vi "UHR-Fleezers Control (host) - 12.6.vi"() -> ()   [LabVIEW 2012] (continued)
  out "X RF Frequency Limits (MHz)":T16={"Minimum"=60.0, "Maximum"=90.0, "Increment"=1.0}
  out "Y RF Frequency Limits (MHz)":T16={"Minimum"=0.0, "Maximum"=40.0, "Increment"=1.0}
  out "Y RF Amplitude Limits (%)":T16={"Minimum"=0.0, "Maximum"=50.0, "Increment"=1.0}
  in  "Manip. X?":bool=TRUE
  in  "Manip. Y?":bool
  in  "Force Manip Abort":bool
  out "Read cal error":errorcluster
  in  "DAQ Delay (ms)":u32=1000
  in  "Start Scan":bool
  in  "Scan axis":bool=TRUE
  in  "Osc. amp. (V)":dbl=5.0
  in  "Osc. center (V)":dbl=5.0
  in  "Osc. freq. (Hz) 2":dbl=1.0
  in  "MCL Mode":u16(ring) items=["Manual Positioning", "Sinusoidal Wave", "Linear Scan"]
  in  "Begin (V)":dbl
  in  "End (V)":dbl=10.0
  in  "N Points":dbl=20.0
  in  "Delay to Interlace (s)":dbl
  in  "Delayed Interlace Start":bool
  in  "Read Lateness and Rel Phase":bool=TRUE
  out "Vec Mean of T1 T2":dbl[](array[numeric])=[nan, nan]
  in  "Cal read wait (s)":u32=5
  out "Time tether formed":timestamp=timestamp(3419012832.6319866 s since 1904-01-01)
  in  "Sample Chamber Stage Serial Port":refnum<visa-resource-name>="Sample-Stage-COM1"
  in  "Chemyx Syringe Pump Serial Port":refnum<visa-resource-name>="ASRL3::INSTR"
  in  "Limit Min (MHz)":dbl=10.0 caption="Min (MHz)"
  in  "Limit Max (MHz)":dbl=16.0 caption="Max (MHz)"
  in  "Limits Enable":bool=TRUE caption="Enable"
  out "AI labels":string[](array[string])=["T1 Y", "T1 X", "T1 Sum", "T2 Y", "T2 X", "T2 Sum", "T1 FB X", "T1 FB Sum", "T2 FB X", "T2 FB Sum", "PSD Y", "PSD X", "PSD Y Sum"]
  in  "Save Trap Pos. Data":bool=TRUE
  in  "Lower Ch. Cap.":bool
  in  "Top 3 Harvard Syringe Pump Serial Port":refnum<visa-resource-name>="Top-Pump3-COM4"
  out "Database link":path
  out "connection reference":T17
  out "Trigger Signal":dbl[](graph)
  in  "Fish mask thresh":dbl=0.5
  in  "Normal (on) or masked test (off)":bool=TRUE
  in  "Stop F (pN) (mask)":dbl=1.0
  in  "Osc. freq. (Hz)":dbl=0.25
  # "External fluorescence triggering tests:"
  # "After"
  # "During"
  # "Trap On?"
  # "BD Flow ON?"
  # "Samp Flow ON?"
  # "Trap Trig. Fl.?"
  # "Zero It"
  # "Floor it\n(e.g., hp unwinding)"
  # "1"
  # "2"
  # "Fl. Down"
  # "Fl. Up"
  # "Bead sep"
  # "Trap Display:"
  # "APD Display:"
  # "Data Saving"
  # "DAQ"
  # "Trap Manipulation"
  # "Bead Calibration"
  # "Bottom Pump (#1)"
  # "Central Sample Channels"
  # "Top Pump (#3)"
  # "Rate param is ul/h\nVolume param is ul"
  # "Chemyx Pump 2"
  # "Units: \n1 = ml/m\n2 = ml/h\n3 = ul/m\n4 = ul/h"
  # "X"
  # "Y"
  # "Oscillate Set 1 freq. (debugging)"
  # "BD 1"
  # "BD 2"
  # "Amp switch 1st is disabled in the fpga!\nSeems its also frequency that needs to go first (for all boards tested so far)."
  # "AOD Raster Scan"
  # "Approx. trap separations"
  # "X"
  # "Y"
  # "FPGA\nreading"
  # "DMA\ntransfer"
  # "APD Integration Loop"
  # "APD Gates"
  # "APD 2 (Cy5)"
  # "APD 3 (Cy2)"
  # "APD 1 (Cy3)"
  # "X"
  # "2D"
  # "Y"
  # "1D"
  # "Digital Out Control"
  # "Analog Out Control (Feedback Loop)"
  # "Laser Intensity Analog Input"
  # "Operational note:\n\nUse the digital out control to adjust red laser\ntiming (fine tuning).\n\nAt the moment, the red laser analog out\ncontrol timing is identical and set by green \nlaser AO timing (in the same loop).  Otherwise\nyou can not get synchronous timing with the\ncurrent AO expansion board.\n\nSimilarly, the AI measurement is also \nsimultaneous for all three lasers (for the same\nreason).\n\nThese controls are kept for possible future\nuse."
  # "Analog Out Control (Feedback Loop)"
  # "Digital Out Control"
  # "Laser Intensity Analog Input"
  # "Operational note:\n\nThe AI measurement is simultaneous for all three lasers\n(see red laser note).\n\nThese controls are kept for possible future use."
  # "Analog Out Control (Feedback Loop)"
  # "Laser Intensity Analog Input"
  # "Digital Out Control"
  # "Total AI Rates (NOT rates/trap)"
  # "(Samples/trap x Trap Sets)"
  # "(Samples/channel x\n8 if averaging (8 channels)\n4 if no averaging)"
  # "Trap 1"
  # "Trap 2"
  # "Flour./Trap 3"
  # "External Video Window"
  # "MCL Position Debugging"
  # "Temporary Control Storage\n(these used to be somewhere else, still want to keep them)"
  # "Database config"
  # "Y"
  # "X"
  # "Trap Position Difference Limits"
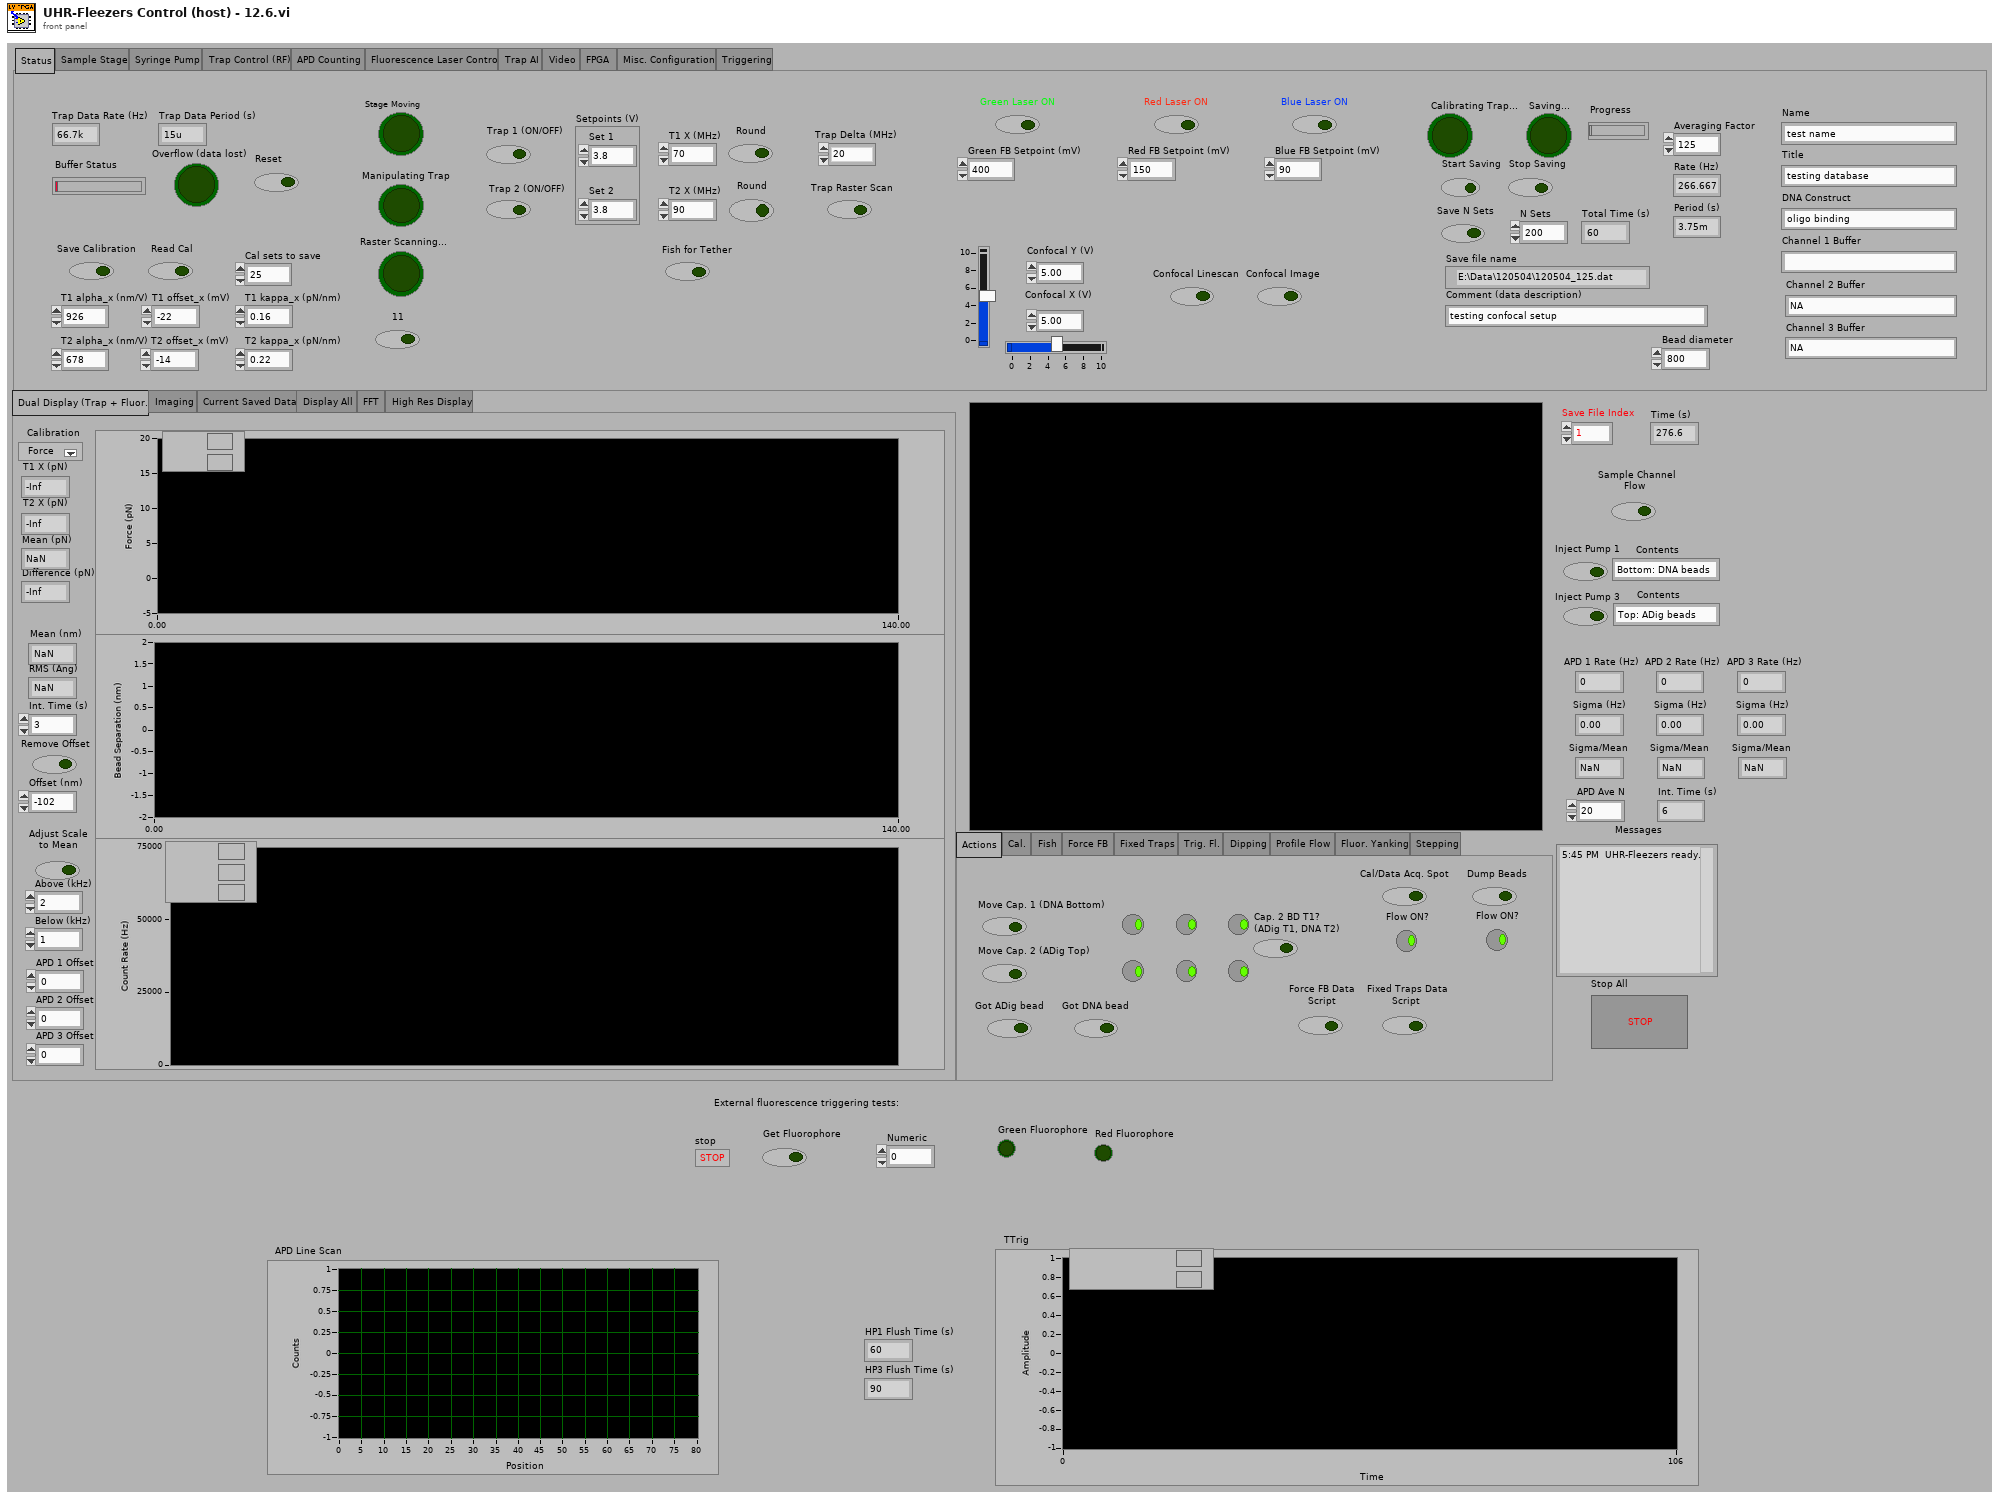
[diagram p1: front panel]
types:
  T1 = enum32{"Actions", "Cal.", "Fish", "Force FB", "Fixed Traps", "Trig. Fl.", "Dipping", "Profile Flow", "Fluor. Yanking", "Stepping"}
  T2 = typedef "IMAQ Image.ctl" = refnum<image>
  T3 = enum32{"Dual Display (Trap + Fluor.)", "Imaging", "Current Saved Data", "Display All", "FFT", "High Res Display"}
  T4 = enum32{"Status", "Sample Stage", "Syringe Pump", "Trap Control (RF)", "APD Counting", "Fluorescence Laser Control", "Trap AI", "Video", "FPGA", "Misc. Configuration", "Triggering"}
  T5 = cluster{"Pump 1":cluster{"Diameter (mm)":dbl, "Units":dbl, "Volume":dbl, "Rate":dbl}, "Pump 2":cluster{"Diameter (mm)":dbl, "Units":dbl, "Volume":dbl, "Rate":dbl}, "Pump 3":cluster{"Diameter (mm)":dbl, "Units":dbl, "Volume":dbl, "Rate":dbl}}
  T6 = enum32{"IR Laser Interlacing (Direct RF Board Control Method)", "AOD Raster Scan", "Feedback on Trap Intensity", "Feedback on Trap Position"}
  T7 = typedef "LVPoint32TypeDef.ctl" = cluster{"Horizontal":i32, "Vertical":i32}
  T8 = cluster{"Scan Range AOD (nm) 2":dbl, "Step Size AOD (nm) 2":dbl, "Scan Speed AOD (nm/s) 2":dbl, "Number of scans (AOD) 2":u16, "Label":string}[]
  T9 = cluster{"proportional gain (Kc)":i16, "integral gain (Kc*Ts/Ti)":i16, "derivative gain (Kc*Td/Ts)":i16}
  T10 = cluster{"Trap 1":fxp<+/-,16,1>, "Trap 2":fxp<+/-,16,1>}
  T11 = cluster{"proportional gain (Kc)":fxp<+/-,16,8>, "integral gain (Kc*Ts/Ti)":fxp<+/-,16,8>, "derivative gain (Kc*Td/Ts)":fxp<+/-,16,8>}
  T12 = cluster{"output high":fxp<+/-,16,1>, "output low":fxp<+/-,16,1>}
  T13 = cluster{"Set 1":fxp<+/-,16,1>, "Set 2":fxp<+/-,16,1>}
  T14 = enum32{"Main Controls", "Green laser (532 nm)", "Red laser (633 nm)", "Blue laser (473 nm)"}
  T15 = cluster{"Set 1":bool, "Set 2":bool, "Set 3":bool}
  T16 = typedef "LVMinMaxIncTypeDef.ctl" = cluster{"Minimum":dbl, "Maximum":dbl, "Increment":dbl}
  T17 = typedef "NI_Database_API.lvlib/Conn ObjectReference.ctl" = refnum<k1>
  T18 = typedef "Image Type" = u32
  T19 = typedef "nirio_resource_hc.ctl" = tag
  T20 = typedef "openfpgaref.8.6.ctl" = refnum<k20>
  T21 = enum16{"empty", "write", "read oldest (queue)", "read newest (stack)", "read all"}
  T22 = cluster{"New Image":T2, "New Image":T2, "New Image":T2, "New Image":T2, "New Image":T2}
  T23 = typedef "XDNodeRunTimeDep.lvlib/timing_clust.ctl" = cluster{"Expected End [f-1]":u64, "Actual End [f-1]":u64, "Finished Late? [f-1]":bool, "Expected End [i-1]":u64, "Actual End [i-1]":u64, "Finished Late? [i-1]":bool, "Expected Start [i]":u64, "Actual Start [i]":u64, "Expected Start [f]":u64, "Actual Start [f]":u64, "Source Name":string, "Structure Name":string, "Period":i64, "Deadline":i64, "Offset":i64, "Start":i64, "Priority":i32, "Timeout":i32, "Mode":T24, "Wakeup Reason":T25, "Error":errorcluster, "Source Type":string, "Secondary Source Type":string, "Global End Time":u64, "Global Start Time":u64, "Frame Duration":u64, "Iteration Duration":u64, "Assigned CPU":i32, "I/O Scan Engine Mode":u32}
  T24 = typedef "XDNodeRunTimeDep.lvlib/nitl_modes.ctl" = enum32{"No Change", "Process missed periods, maintain original phase", "Discard missed periods, maintain original phase", "Process missed periods, ignore original phase", "Discard missed periods, ignore original phase"}
  T25 = typedef "XDNodeRunTimeDep.lvlib/wakeup.ctl" = enum32{"Normal", "Aborted", "Asynchronous wakeup", "Timing source error", "Timed loop error", "Timeout"}
  T26 = enum32{"Status", "Sample Stage", "Syringe Pump", "Trap Control (RF)", "APD Counting", "Fluorescence Laser Control", "Trap AI", "Video", "FPGA"}
  T27 = enum32{"Status", "Sample Stage", "Syringe Pump", "Trap Control (RF)", "APD Counting", "Fluorescence Laser Control", "Trap AI", "Video", "FPGA", "Misc. Configuration"}
  T28 = enum16{"big-endian, network order", "native, host order", "little-endian"}
  T29 = enum16{"open", "replace", "create", "open or create", "replace or create", "replace or create with confirmation"}
  T30 = cluster{"Scan Range AOD (nm) 2":dbl, "Step Size AOD (nm) 2":dbl, "Scan Speed AOD (nm/s) 2":dbl, "Number of scans (AOD) 2":u16, "Label":string}
  T31 = cluster{"[0]":dbl, "[1]":dbl, "[2]":dbl, "[3]":dbl, "[4]":dbl, "[5]":dbl}
  T32 = cluster{"Diameter (mm)":dbl, "Units":dbl, "Volume":dbl, "Rate":dbl}
  T33 = cluster{"Left":i32, "Top":i32, "Width":u32, "Height":u32}
  T34 = cluster{cluster{"Left":i32, "Top":i32, "Width":u32, "Height":u32}}[]
  T35 = enum32{"Normal Display", "Dual Display (APD)", "FFT", "High Res Display"}
  T36 = cluster{"Origin Pixel":cluster{"X":sgl, "Y":sgl}, "Angle Relative to Horizontal (deg)":sgl, "Axis Reference":u32}
  T37 = typedef "Simple Grid Descriptor" = cluster{"X Step":sgl, "Y Step":sgl, "Unit":T38}
  T38 = typedef "Image Unit" = enum32{"Undefined", "Angström", "Micrometer", "Millimeter", "Centimeter", "Meter", "Kilometer", "Microinch", "Inch", "Feet", "Nautical miles", "Standard miles", "Steps"}
  T39 = cluster{"averaging mode":u16, "weighting mode":u16, "number of averages":u32}
  T40 = cluster{"dB On (F)":bool, "unwrap phase (F)":bool, "convert to degree (F)":bool}
  T41 = cluster{string, string, string, string, string, string, string, string}
  T42 = cluster{string, string, string, string, string, string, string, string, string, string, string, string}
  T43 = cluster{string, string, string, string, string, string, string, string, string, string, string, string, string}
  T44 = cluster{string, string, string, string, string, string, string, string, string, string, string, string, string, string}
  T45 = cluster{"BD 1 Frequency 1 (MHz)":dbl, "BD 1 Frequency 2 (MHz)":dbl}
  T46 = cluster{"f0":dbl, "df":dbl, "magnitude":dbl[]}[][]
  T47 = cluster{"Comment (data description)":string, "Channel 1 Buffer":string, "Channel 2 Buffer":string, "Channel 3 Buffer":string, "Title":string, "DNA Construct":string, "Bead diameter":dbl, "Name":string}
  T48 = enum32{"setting", "request", "request control", "info", "statistics", "system settings", "I/O sub system", "HRT control", "camera descriptions", "device specific data", "event sub system settings", "event sub system results", "image memory manager"}
  T49 = typedef "AviRefnum.ctl" = refnum<k1>
  T50 = typedef "imagedata.ctl" = cluster{"image type":i32, "image depth":i32, "image":u8[], "mask":u8[], "colors":u32[], "Rectangle":cluster{"left":i16, "top":i16, "right":i16, "bottom":i16}}
diagram:
  w6 = u16 10 items=["1.0"=10, "1.5"=15, "2.0"=20] ("stop bits (10: 1 bit)")
  w73 = u16 20 items=["1.0"=10, "1.5"=15, "2.0"=20] ("stop bits (10: 1 bit)")
  w76 = u16 20 items=["1.0"=10, "1.5"=15, "2.0"=20] ("stop bits (10: 1 bit)")
  w102 = u16 20 items=["1.0"=10, "1.5"=15, "2.0"=20] ("stop bits (10: 1 bit)")
  w12 = T18 2 items=["Grayscale (U8)", "Grayscale (I16)", "Grayscale (SGL)", "Complex (CSG)", "RGB (U32)", "HSL (U32)", "RGB (U64)", "Grayscale (U16)"] ("Image Type")
  w232 = 10.0 ("y")
  w231 = 32767.0 ("y")
  w247 = 6.0  # clock mult.
  w248 = 49152000.0  # TCXO frequ.
  # "What are these?"
  # "I don't think you need to do this.\nEverytime you want to adjust phase you always set this anyway.\nSince we removed the separate +/- controls.\n\nHaven't added for added fl lasers.  Should remove this code."
  # "Bottom 1 Harvard"
  # "Top 3 Harvard"
  # "Center Harvard"
  # "Bottom 1 Harvard"
  # "Top 3 Harvard"
  # "Center Harvard"
  n1 = Build Array("DIO count 1 (ticks)", "DIO count 2 (ticks)", "DIO count 3 (ticks)") -> (w153:u16[])
  n2 = xnode "Open FPGA VI Reference"("resource name"=T19 "750kHzDAQ") -> ("FPGA VI Reference Out"=w256:T20, "error out"=w255:errorcluster)  [unwired: 1 in]
  n3 = local read "AO1"() -> (w226:dbl)
  n4 = local read "AO2"() -> (w225:dbl)
  n5 = local read "Scan Increment (MHz)"() -> (w243:dbl)
  n6 = local read "Continuous MCL Scanning"() -> (w213:bool)
  n7 = local read "Fast Scan Dir"() -> (w212:bool)
  n8 = xnode "Invoke Method"("FPGA VI Reference In"=w256, "error in"=w255) -> ("FPGA VI Reference Out"=w16:T20, "error out"=w172:errorcluster)
  n9 = local read "Number of scans (MCL)"() -> (w214:u64)
  n10 = Multiply(x=w226, y=w231) -> (x*y=w228:dbl)
  n11 = Multiply(x=w225, y=w231) -> (x*y=w230:dbl)
  n12 = Divide(x=w228, y=w232) -> (x/y=w227:dbl)
  n13 = Divide(x=w230, y=w232) -> (x/y=w229:dbl)
  n14 = To Word Integer(number=w227) -> (16bit integer=w224:i16)
  n15 = To Word Integer(number=w229) -> (16bit integer=w223:i16)
  n16 = Not(x=w212) -> (.not. x?=w207:bool)
  n17 = local read "Cycles/step (MCL)"() -> (w215:u64)
  n18 = Multiply(x=w243, y=1000.0) -> (x*y=w250:dbl)
  n19 = local read "Scan steps (MCL)"() -> (w216:u64)
  n20 = local read "Desired Scan Incr (V)"() -> (w218:dbl)
  n21 = Scale By Power Of 2(n=48, x=w250) -> (x*2^n=w251:dbl)
  n22 = Unbundle By Name(cluster{"output high":i16, "output low":i16} {"output high"=3000, "output low"=0} ("FB output range 1")) -> ("output high"=w54:i16, "output low"=w53:i16)
  n23 = Multiply(x=w248, y=w247) -> (x*y=w246:dbl)
  n24 = Divide(x=w251, y=w246) -> (x/y=w245:dbl)
  n25 = local read "Setpoints (V)"() -> (w262:cluster{"Set 1":dbl, "Set 2":dbl})
  n26 = To Quad Integer(1:w245) -> (0:w242:i64)
  n27 = Divide(x=40000000.0, y="AI Count (ticks)") -> (x/y=w203:dbl)
  n28 = Multiply(x=w218, y=32767.0) -> (x*y=w220:dbl)
  n29 = local read "Trap Intensity PID Gains"() -> (w257:T9)
  n30 = local write "Trap Pos FIFO Timeout"(u16 0 ("Trap Pos FIFO Timeout")) -> ()
  n31 = local read "Number Interlace Sets"() -> (w146:u8)
  n32 = Split 1D Array(array=w153, index=w146) -> (first subarray=w155:u16[])  [unwired: 1 out]
  n33 = Add Array Elements(numeric array=w155) -> (sum=w154:u16)
  n34 = local read "# Samples/channel"() -> (w235:u32)
  n35 = local read "Number of F/B Scans (AOD)"() -> (w236:u16)
  n36 = local read "Not-Interlacing Set"() -> (w145:enum32{"Set 1", "Set 2", "Set 3"})
  n37 = To Unsigned Byte Integer(number=w145) -> (unsigned 8bit integer=w151:u8)
  n38 = Index Array(array=w153, index=w151) -> (element=w152:u16)
  n39 = local read "Feedback On/Off"() -> (w265:cluster{"Set 1":bool, "Set 2":bool})
  n40 = local read "Scan steps (AOD)"() -> (w241:u64)
  n41 = local read "All FB On/Off"() -> (w266:bool)
  n42 = local read "Cycles/step (AOD)"() -> (w240:u64)
  n43 = local write "AI rate (Hz)"(w203) -> ()
  n44 = Divide(x=w220, y=10.0) -> (x/y=w219:dbl)
  n45 = Multiply(x=w241, y=w240) -> (x*y=w239:u64)
  n46 = Unbundle By Name(w257) -> ("proportional gain (Kc)"=w58:i16, "integral gain (Kc*Ts/Ti)"=w57:i16, "derivative gain (Kc*Td/Ts)"=w56:i16)
  n47 = property on="AI Count (ticks)" class="DigNum (strict)"("Val(Sgnl)"="AI Count (ticks)") -> ()  [unwired: 2 in, 2 out]
  n48 = Multiply(x=3276.7, y=w262) -> (x*y=w261:cluster{"Set 1":dbl, "Set 2":dbl})
  n49 = To Word Integer(number=w219) -> (16bit integer=w217:i16)
  n50 = Multiply(x=w239, y=u64 2) -> (x*y=w237:u64)
  n51 = Divide(x=w203, y="FPGA Ave.") -> (x/y=w204:dbl)
  n52 = To Word Integer(number=w261) -> (16bit integer=w260:cluster{"Set 1":i16, "Set 2":i16})
  n53 = Multiply(x=w237, y=w236) -> (x*y=w234:u64)
  n54 = local read "Sets to FIFO (Traps)"() -> (w62:T15)
  n55 = local write "Ave. Rate (Hz)"(w204) -> ()
  n56 = Divide(x=w234, y=w235) -> (x/y=w233:dbl)
  n57 = Unbundle By Name(w260) -> ("Set 1"=w259:i16, "Set 2"=w258:i16)
  n58 = local read "2D or 1D Scan"() -> (w164:bool)
  n59 = local write "Data points/scans"(w234) -> ()
  n60 = local read "Scan BD"() -> (w252:bool)
  n61 = And(x=w265, y=w266) -> (x .and. y?=w264:cluster{"Set 1":bool, "Set 2":bool})
  n62 = local write "Data points/scan (f/b)"(w237) -> ()
  n63 = Reciprocal(x=w204) -> (1/x=w205:dbl)
  n64 = local read "N Acq Sets (Traps + Fl.)"() -> (w196:i16)
  n65 = local write "N sets should be saved"(w233) -> ()
  n66 = Unbundle By Name(w264) -> ("Set 1"=w268:bool, "Set 2"=w267:bool)
  n67 = local read "Interlace"() -> (w147:bool)
  n68 = Select(t=w154, s=w147, f=w152) -> (s? t:f=w144:u16)
  n69 = local write "Update Count (MCL)"(w144) -> ()
  n70 = local write "Total Counts (ticks)"(w144) -> ()
  n71 = local write "Ave. Period (s)"(w205) -> ()
  n72 = Unbundle By Name(w62) -> ("Set 1"=w61:bool, "Set 2"=w60:bool, "Set 3"=w59:bool)
  n73 = property on="2D or 1D Scan" class="Bool (strict)"("Val(Sgnl)"=w164) -> ()  [unwired: 2 in, 2 out]
  n74 = xnode "Read/Write Control"("FPGA VI Reference In"=w163, "error in"=w172, "ai count"="AI Count (ticks)", "Interlace ON/OFF"=w147, "Number Interlace Cycles"=w146, "Set 1"=w61, "Set 2"=w60, "Set 3"=w59, "FB On/Off Set 1"=w268, "FB On/Off Set 2"=w267, "Interlace Off Parameters"=w145, "FB Setpoint Set 1"=w259, "FB Setpoint Set 2"=w258, "P1"=w58, "I1"=w57, "D1"=w56, "FB1 output high"=w54, "FB1 output low"=w53, "Cycles per step"=w240, "Scan BD"=w252, "Number of scans"=w236, "Scan steps"=w241, "Scan freq.  increment"=w242, "AO1"=w224, "AO2"=w223, "Scan freq.  increment (MCL)"=w217, "Scan steps (MCL)"=w216, "Cycles per step (MCL)"=w215, "Number of scans (MCL)"=w214, "MCL count"=w144, "Cont. Scan (MCL)"=w213, "MCL Scan Axis"=w207, "1D or 2D Scan?"=w164, "N of AI1 Int Acq Sets"=w196, "Amp switch delay"="Amp switch delay", "Swap F1 and F2"="Swap F1 and F2", "APD to FIFO"=FALSE, "DIO count 1 (ticks)"="DIO count 1 (ticks)", "DIO count 2 (ticks)"="DIO count 2 (ticks)", "DIO count 3 (ticks)"="DIO count 3 (ticks)") -> ("FPGA VI Reference Out"=w18:T20, "error out"=w17:errorcluster)  [unwired: 1 in]
  n75 = local read "Laser interlacing mode"() -> (w143:enum32{"Laser ON", "Laser OFF", "Interlace"})
  n76 = local read "Green Laser ON"() -> (w142:bool)
  n77 = local read "Trap Pos. FB Range"() -> (w52:T12)
  n78 = local read "Trap Pos. FB Gains"() -> (w51:T11)
  n79 = Multiply(x="Green Intensity % (FB OFF)", y=655.35) -> (x*y=w135:dbl)
  n80 = local read "Invert laser interlacing"() -> (w31:bool)
  n81 = local read "Trap Pos. AI1 X Pre-scale"() -> (w90:u16)
  n82 = Multiply(x="Green FB Setpoint (mV)", y=3.2767) -> (x*y=w132:dbl)
  n83 = local read "Trap Pos FB Int Count"() -> (w84:u16)
  n84 = local read "Differential FB?"() -> (w78:bool)
  n85 = local read "Neg. TTrig FPGA"() -> (w80:bool)
  n86 = Multiply(x="Red FB Setpoint (mV)", y=3.2767) -> (x*y=w39:dbl)
  n87 = To Unsigned Word Integer(number=w135) -> (unsigned 16bit integer=w133:u16)
  n88 = Multiply(x="Red Intensity % (FB OFF)", y=655.35) -> (x*y=w35:dbl)
  n89 = To Word Integer(number=w132) -> (16bit integer=w130:i16)
  n90 = Unbundle By Name("Green FB Gains") -> ("proportional gain (Kc)"=w43:i16, "integral gain (Kc*Ts/Ti)"=w42:i16, "derivative gain (Kc*Td/Ts)"=w41:i16)
  n91 = Unbundle By Name("Red FB Gains") -> ("proportional gain (Kc)"=w28:i16, "integral gain (Kc*Ts/Ti)"=w27:i16, "derivative gain (Kc*Td/Ts)"=w26:i16)
  n92 = case shown="False" w142 {
    tunnel: w143 -> [_ w294]
    tunnel: [enum32{"Laser ON", "Laser OFF", "Interlace"}."Laser OFF" ("Green laser mode") w294] -> w30
    frame False {
    }
    frame True {
    }
  }
  n93 = To Word Integer(number=w39) -> (16bit integer=w36:i16)
  n94 = Unbundle By Name(w51) -> ("proportional gain (Kc)"=w47:fxp<+/-,16,8>, "integral gain (Kc*Ts/Ti)"=w46:fxp<+/-,16,8>, "derivative gain (Kc*Td/Ts)"=w45:fxp<+/-,16,8>)
  n95 = To Unsigned Word Integer(number=w35) -> (unsigned 16bit integer=w32:u16)
  n96 = Unbundle By Name(w52) -> ("output high"=w50:fxp<+/-,16,1>, "output low"=w48:fxp<+/-,16,1>)
  n97 = local read "Trap Pos FB Monitor\nT1 or T2"() -> (w95:bool)
  n98 = local read "Trap Pos FB Negate Action"() -> (w94:bool)
  n99 = local read "Trap Pos. FB Offset Factor"() -> (w93:i64)
  n100 = local read "Trap Pos. FB Mult Factor"() -> (w92:i64)
  n101 = xnode "Read/Write Control"("FPGA VI Reference In"=w18, "error in"=w17, "Invert GI 2"=w31, "Operating Mode 2"=w30, "P3"=w43, "I3"=w42, "D3"=w41, "Green FB Setpoint"=w130, "Green FB On/Off"="Green FB On/Off", "Current Out"=w133, "Green int current ON count adj"="Green int current ON count adj", "Operating Mode"=w30, "Invert GI"=w31, "Trap Pos FB Monitor T1 or T2"=w95, "Trap Pos FB Negate Action"=w94, "Trap Pos. FB Offset Factor"=w93, "Trap Pos. FB Mult Factor"=w92, "Force feedback"=FALSE, "AI1 X Scale"=w90, "Trap Pos to FIFO"=TRUE, "Trap Pos FB Int Count"=w84, "TTrig Negate Pos"=w80, "FB Trig Integrate"="FB Trig Integrate", "Diff FB Measurement?"=w78, "Negate Diff?"="Negate Diff?", "P2"=w47, "I2"=w46, "D2"=w45, "FB2 output high"=w50, "FB2 output low"=w48, "Red FB Setpoint"=w36, "RI Current Out"=w32, "Red Laser Operating Mode"=w30, "RI Operating Mode 2"=w30, "Invert RI 2"=w31, "Invert RI"=w31, "P4"=w28, "I4"=w27, "D4"=w26, "Red FB On/Off"="Red FB On/Off") -> ("FPGA VI Reference Out"=w22:T20, "error out"=w24:errorcluster)
  n102 = stacked-sequence {
    tunnel: w24 -> [_ _ _ w305]
    tunnel: [_ _ _ w305] -> w23
    tunnel: w22 -> [_ _ _ w306]
    tunnel: [_ _ _ w306] -> w21
    frame #0 {
      w295 = T21."empty" ("mode")
      # "Clear external fluorescence triggering FIFO"
      # "APD loop counts"
      # "Fluorescence loop counts (rates)"
      n103 = local read "APD Integration Time (s)"() -> (w297:dbl)
      n104 = local read "Interlace ON count"() -> (w298:u16)
      n105 = call "Smart Buffer (DBL) 1.vi"("mode"=w295) -> ()  [unwired: 5 in, 6 out]
      n106 = call "Smart Buffer (DBL) 2.vi"("mode"=w295) -> ()  [unwired: 5 in, 6 out]
      n107 = property on="APD Integration Time (s)" class="DigNum (strict)"("Val(Sgnl)"=w297) -> ()  [unwired: 2 in, 2 out]
      n108 = property on="Interlace ON count" class="DigNum (strict)"("Val(Sgnl)"=w298) -> ()  [unwired: 2 in, 2 out]
      "Number of APDs" <- 3.0 ("Number of APDs")
    }
    frame #1 {
      # "Number of APDs affects\nAPD DMA transfer"
      # "General settings for all lasers:"
      # "And includes all laser\nON/OFF settings"
      # "Fluorescent lasers settings:"
      # "Blue laser settings:"
      n109 = local read "Laser interlacing mode"() -> (w300:enum32{"Laser ON", "Laser OFF", "Interlace"})
      n110 = local read "Invert laser interlacing"() -> (w299:bool)
      n111 = local read "Blue FB On/Off"() -> (w301:bool)
      n112 = property on="Blue FB On/Off" class="Bool (strict)"("Val(Sgnl)"=w301) -> ()  [unwired: 2 in, 2 out]
      n113 = property on="Invert laser interlacing" class="Bool (strict)"("Val(Sgnl)"=w299) -> ()  [unwired: 2 in, 2 out]
      n114 = property on="Laser interlacing mode" class="RadioBtnsControl (strict)"("Val(Sgnl)"=w300) -> ()  [unwired: 2 in, 2 out]
    }
    frame #2 {
      w302 = path "C:/Home/wheeler/Comstock-LabView-Link.udl" ("connection information")
      # "Initialize the database connection"
      n115 = call-poly <vilib>:"DB Tools Open Connection.vi"("connection information"=w302) -> ("connection reference"=w303:T17)  [unwired: 7 in, 1 out]
      "connection reference" <- w303
      n116 = local write "connection reference"(w303) -> ()
      n117 = local write "Database link"(w302) -> ()
    }
    frame #3 {
      n118 = Wait (ms)(milliseconds to wait=u32 1000) -> ()  [unwired: 1 out]
    }
  }
  n119 = local write "Offset (nm)"(0.0 ("Offset (nm)")) -> ()
  n120 = local write "Bead Mean (nm)"(0.0 ("Bead Mean (nm)")) -> ()
  n121 = case shown="\"2axisAOD\"" "1axis AOM vs 2 axis AOD" {
    tunnel: [T16 {"Minimum"=0.0, "Maximum"=40.0, "Increment"=1.0} ("Min Max Inc") T16 {"Minimum"=60.0, "Maximum"=90.0, "Increment"=1.0} ("Min Max Inc")] -> w3
    tunnel: [T16 {"Minimum"=0.0, "Maximum"=45.0, "Increment"=1.0} ("Data Entry Limits") T16 {"Minimum"=0.0, "Maximum"=50.0, "Increment"=1.0} ("Data Entry Limits")] -> w1
    frame "2axisAOD" {
      # "Amp Limits"
      # "Freq Limits"
    }
    frame "1axis", Default {
      # "Amp Lmits"
      # "Freq Limits"
    }
  }
  n122 = xnode "Invoke Method"("FPGA VI Reference In"=w21, "error in"=w23, "Requested Depth"="Trap AI FIFO Depth") -> ("FPGA VI Reference Out"=w98:T20, "error out"=w97:errorcluster)  [unwired: 1 out]
  n123 = xnode "Invoke Method"("FPGA VI Reference In"=w98, "error in"=w97, "Requested Depth"="Trap Position FIFO Depth") -> ("FPGA VI Reference Out"=w86:T20, "error out"=w85:errorcluster)  [unwired: 1 out]
  n124 = flat-sequence "Safety limits on RF frequencies and amplitudes (for AOM protection)" {
    tunnel: w16 -> [w315]
    tunnel: [w315] -> w163
    tunnel: [w312] -> w162
    tunnel: [w311] -> w161
    tunnel: [w313] -> w159
    tunnel: [w314] -> w160
    tunnel: w3 -> [w312]
    tunnel: w1 -> [w311]
    frame #0 {
      w314 = T16 {"Minimum"=0.0, "Maximum"=40.0, "Increment"=1.0} ("Min Max Inc")
      w313 = T16 {"Minimum"=0.0, "Maximum"=45.0, "Increment"=1.0} ("Data Entry Limits")
      n125 = property on="BD 2 Frequency 1 (MHz)" class="DigNum (strict)"("Data Range"=w314) -> ()  [unwired: 2 in, 2 out]
      n126 = property on="BD 2 Frequency 3 (MHz)" class="DigNum (strict)"("Data Range"=w314) -> ()  [unwired: 2 in, 2 out]
      n127 = property on="BD 2 Frequency 2 (MHz)" class="DigNum (strict)"("Data Range"=w314) -> ()  [unwired: 2 in, 2 out]
      n128 = property on="BD 1 Frequency 1 (MHz)" class="DigNum (strict)"("Data Range"=w312) -> ()  [unwired: 2 in, 2 out]
      n129 = property on="BD 1 Frequency 2 (MHz)" class="DigNum (strict)"("Data Range"=w312) -> ()  [unwired: 2 in, 2 out]
      n130 = property on="BD 1 Frequency 3 (MHz)" class="DigNum (strict)"("Data Range"=w312) -> ()  [unwired: 2 in, 2 out]
      n131 = property on="BD 2 Amplitude 1 (%)" class="DigNum (strict)"("Data Range"=w313) -> ()  [unwired: 2 in, 2 out]
      n132 = property on="BD 2 Amplitude 2 (%)" class="DigNum (strict)"("Data Range"=w313) -> ()  [unwired: 2 in, 2 out]
      n133 = property on="BD 2 Amplitude 3 (%)" class="DigNum (strict)"("Data Range"=w313) -> ()  [unwired: 2 in, 2 out]
      n134 = property on="BD 1 Amplitude 3 (%)" class="DigNum (strict)"("Data Range"=w311) -> ()  [unwired: 2 in, 2 out]
      n135 = property on="BD 1 Amplitude 2 (%)" class="DigNum (strict)"("Data Range"=w311) -> ()  [unwired: 2 in, 2 out]
      n136 = property on="BD 1 Amplitude 1 (%)" class="DigNum (strict)"("Data Range"=w311) -> ()  [unwired: 2 in, 2 out]
      "X RF Frequency Limits (MHz)" <- w312
      "X RF Amplitude Limits (%)" <- w311
      "Y RF Amplitude Limits (%)" <- w313
      "Y RF Frequency Limits (MHz)" <- w314
    }
  }
  n137 = xnode "Invoke Method"("FPGA VI Reference In"=w86, "error in"=w85) -> ("FPGA VI Reference Out"=w171:T20, "error out"=w170:errorcluster)  [unwired: 1 in]
  n138 = flat-sequence "Initial FPGA Loop Relative Phase Adjustment" {
    tunnel: "Initial Phase Adjustment (AI1)" -> [w330]
    tunnel: "Initial Phase Adjustment (GI)" -> [w329]
    tunnel: w171 -> [w328]
    tunnel: w170 -> [w327]
    tunnel: "Initial Phase Adj. (MCL)" -> [w326]
    tunnel: [w331] -> w180
    tunnel: [w325] -> w176
    tunnel: "Initial Phase Adjustment (APD Acq)" -> [w324]
    tunnel: "Initial Phase Adjustment (APD 1 Gate)" -> [w323]
    tunnel: "Initial Phase Adjustment (Green FB)" -> [w322]
    tunnel: "Initial Phase Adjustment (GI) 2" -> [w321]
    tunnel: "Initial Phase Adjustment (APD 2 Gate)" -> [w320]
    tunnel: "Initial Phase Adjustment (RI)" -> [w319]
    tunnel: "Initial Phase Adjustment (BI DO)" -> [w318]
    tunnel: "Initial Phase Adjustment (BI AO)" -> [w317]
    tunnel: "Initial Phase Adjustment (APD 3 Gate)" -> [w316]
    tunnel: w180 -> [w333]
    tunnel: [w334] -> w177
    tunnel: w176 -> [w334]
    tunnel: [w333] -> w175
    tunnel: w177 -> [w337]
    tunnel: w175 -> [w336]
    tunnel: [w339] -> w174
    tunnel: [w338] -> w173
    tunnel: [w341] -> w178
    tunnel: [w342] -> w179
    tunnel: w174 -> [w342]
    tunnel: w173 -> [w341]
    frame #0 {
      n139 = xnode "Read/Write Control"("FPGA VI Reference In"=w328, "error in"=w327, "Phase count adjustment"=w330, "Phase count adjustment (GI)"=w329, "Phase count adjustment (MCL)"=w326, "Phase Count Adjustment (APD Acq)"=w324, "Phase count adjustment (APD 1 Gate)"=w323, "Phase count adjustment (APD 2 Gate)"=w320, "Phase count adjustment (Green FB)"=w322, "Phase count adjustment (GI) 2"=w321, "Phase count adjustment (RI)"=w319, "Phase count adjustment (BI AO)"=w317, "Phase count adjustment (BI D)"=w318, "Phase count adjustment (APD 3 Gate)"=w316) -> ("FPGA VI Reference Out"=w325:T20, "error out"=w331:errorcluster)
    }
    frame #1 {
      n140 = Wait (ms)(milliseconds to wait=u32 100) -> ()  [unwired: 1 out]
    }
    frame #2 {
      w335 = TRUE
      n141 = xnode "Read/Write Control"("FPGA VI Reference In"=w337, "error in"=w336, "+ phase"=w335, "+ phase (GI)"=w335, "+ phase (MCL)"=w335, "+ phase (APD Acq)"=w335, "+ phase (APD 1 Gate)"=w335, "+ phase (APD 2 Gate)"=w335, "+ phase (Green FB)"=w335, "+ phase (GI) 2"=w335, "+ phase (RI)"=w335, "+ phase (BI AO)"=w335, "+ phase (BI D)"=w335, "+ phase (APD 3 Gate)"=w335) -> ("FPGA VI Reference Out"=w338:T20, "error out"=w339:errorcluster)
    }
    frame #3 {
      n142 = Wait (ms)(milliseconds to wait=u32 100) -> ()  [unwired: 1 out]
    }
  }
  n143 = local read "Phase adj. (Green FB)"() -> (w156:i16)
  n144 = local read "Phase adj. (GI) 2"() -> (w136:i16)
  n145 = local read "Phase adjust (MCL)"() -> (w208:i16)
  n146 = local read "Phase adj. (AI1)"() -> (w210:i16)
  n147 = local read "Phase adj. (GI)"() -> (w209:i16)
  n148 = xnode "Read/Write Control"("FPGA VI Reference In"=w178, "error in"=w179, "Phase count adjustment"=w210, "Phase count adjustment (GI)"=w209, "Phase count adjustment (MCL)"=w208, "Phase Count Adjustment (APD Acq)"="Phase Adj. (APD Acq)", "Phase count adjustment (APD 1 Gate)"="Phase Adj. (APD 1 Gate)", "Phase count adjustment (APD 2 Gate)"="Phase Adj. (APD 2 Gate)", "Phase count adjustment (Green FB)"=w156, "Phase count adjustment (GI) 2"=w136) -> ("FPGA VI Reference Out"=w122:T20, "error out"=w185:errorcluster)
  n149 = call "Initialize RF boards - interlace 3.vi"("error in"=w185, "FPGA VI Reference In"=w122) -> ("error out"=w183:errorcluster, "FPGA VI Reference Out"=w184:T20)
  n150 = call "set RF board frequency - interlace.vi"("Board 2 Frequency Limits"=w160, "Board 1 Frequency Limits"=w162, "error in"=w183, "FPGA VI Reference In"=w184, "Board 2 Frequency 3 (MHz)"="BD 2 Frequency 3 (MHz)", "Board 1 Frequency 3 (MHz)"="BD 1 Frequency 3 (MHz)", "Board 2 Frequency 2 (MHz)"="BD 2 Frequency 2 (MHz)", "Board 2 Frequency 1 (MHz)"="BD 2 Frequency 1 (MHz)", "Board 1 Frequency 2 (MHz)"="BD 1 Frequency 2 (MHz)", "Board 1 Frequency 1  (MHz)"="BD 1 Frequency 1 (MHz)") -> ("error out"=w283:errorcluster, "FPGA VI Reference Out"=w284:T20)
  n151 = call "set RF board amplitude - interlace.vi"("Board 2 Amplitude Limits"=w159, "Board 1 Amplitude Limits"=w161, "error in"=w283, "FPGA VI Reference In"=w284, "Board 2 Amplitude 3 (%)"="BD 2 Amplitude 3 (%)", "Board 1 Amplitude 3 (%)"="BD 1 Amplitude 3 (%)", "Board 2 Amplitude 2 (%)"="BD 2 Amplitude 2 (%)", "Board 2 Amplitude 1 (%)"="BD 2 Amplitude 1 (%)", "Board 1 Amplitude 2 (%)"="BD 1 Amplitude 2 (%)", "Board 1 Amplitude 1 (%)"="BD 1 Amplitude 1 (%)") -> ("error out"=w271:errorcluster, "FPGA VI Reference Out"=w272:T20)
  n152 = flat-sequence {
    tunnel: w272 -> [w352]
    tunnel: w271 -> [w351]
    tunnel: [w350] -> w276
    tunnel: [w349] -> w275
    tunnel: [w356] -> w274
    tunnel: w276 -> [w356]
    tunnel: [w355] -> w273
    tunnel: w275 -> [w355]
    tunnel: w274 -> [w365]
    tunnel: w273 -> [w364]
    tunnel: [w363] -> w15
    tunnel: [w362] -> w87
    frame #0 {
      w343 = FALSE ("Retract Pump 3")
      n153 = local read "Trap 1 (ON/OFF)"() -> (w344:bool)
      n154 = xnode "Read/Write Control"("FPGA VI Reference In"=w352, "error in"=w351, "Direct RF Box  Communication"=FALSE) -> ("FPGA VI Reference Out"=w350:T20, "error out"=w349:errorcluster)
      n155 = local write "Saving..."(FALSE ("Saving Data")) -> ()
      n156 = local write "Stop All"(FALSE ("Stop All")) -> ()
      n157 = local write "Retract Pump 1"(w343) -> ()
      n158 = local write "Retract Pump 3"(w343) -> ()
      n159 = local write "Index"(1.0 ("Index")) -> ()
      n160 = property on="Trap 1 ON" class="Bool (strict)"("Value"=w344) -> ()  [unwired: 2 in, 2 out]
      "Manipulating Trap" <- FALSE ("Manipulating Trap")
    }
    frame #1 {
      n161 = local read "Trap 2 (ON/OFF)"() -> (w354:bool)
      n162 = Wait (ms)(milliseconds to wait=u32 10) -> ()  [unwired: 1 out]
      n163 = property on="Trap 2 ON" class="Bool (strict)"("Val(Sgnl)"=w354) -> ()  [unwired: 2 in, 2 out]
    }
    frame #2 {
      n164 = local read "Scan Range (nm)"() -> (w358:dbl)
      n165 = xnode "Read/Write Control"("FPGA VI Reference In"=w365, "error in"=w364, "FPGA Controls  RF Box"=TRUE ("Direct RF Box  Communication")) -> ("FPGA VI Reference Out"=w363:T20, "error out"=w362:errorcluster)
      n166 = call "Update messages.vi"("Message to add"="UHR-Fleezers ready.", "Old message string"="") -> ("New message string"=w361:string)
      n167 = local write "Messages"(w361) -> ()
      n168 = property on="Scan Range (nm)" class="DigNum (strict)"("Val(Sgnl)"=w358) -> ()  [unwired: 2 in, 2 out]
    }
  }
  n169 = Subtract(x="BD 1 Frequency 1 (MHz)", y="BD 1 Frequency 2 (MHz)") -> (x-y=w195:dbl)
  n170 = Subtract(x="BD 2 Frequency 1 (MHz)", y="BD 2 Frequency 2 (MHz)") -> (x-y=w194:dbl)
  n171 = Square(x=w194) -> (x^2=w192:dbl)
  n172 = Square(x=w195) -> (x^2=w193:dbl)
  n173 = Add(x=w193, y=w192) -> (x+y=w191:dbl)
  n174 = Square Root(x=w191) -> (sqrt(x)=w190:dbl)
  n175 = local write "Trap Delta (MHz)"(w190) -> ()
  n176 = call-poly "VISA Configure Serial Port"("VISA resource name"="VISA resource name", "baud rate (9600)"=u32 115200, "stop bits (10: 1 bit)"=w6) -> ("VISA resource name out"=w5:refnum<visa-resource-name>, "error out"=w4:errorcluster)  [unwired: 4 in, 7 out]
  n177 = call-poly "VISA Configure Serial Port"("VISA resource name"="Bottom  1 Harvard Syringe Pump Serial Port", "baud rate (9600)"=u32 115200, "stop bits (10: 1 bit)"=w73) -> ("VISA resource name out"=w69:refnum<visa-resource-name>, "error out"=w68:errorcluster)  [unwired: 4 in, 7 out]
  n178 = call-poly "VISA Configure Serial Port"("VISA resource name"="Top 3 Harvard Syringe Pump Serial Port", "baud rate (9600)"=u32 115200, "stop bits (10: 1 bit)"=w76) -> ("VISA resource name out"=w71:refnum<visa-resource-name>, "error out"=w70:errorcluster)  [unwired: 4 in, 7 out]
  n179 = call-poly "VISA Configure Serial Port"("VISA resource name"="Sample Chamber Stage Serial Port") -> ("VISA resource name out"=w117:refnum<visa-resource-name>, "error out"=w118:errorcluster)  [unwired: 5 in, 8 out]
  "Stage Control Serial Error" <- w118
  n180 = local write "Blue Error Out"(w4) -> ()
  n181 = call-poly "VISA Configure Serial Port"("VISA resource name"="Center Harvard Syringe Pump Serial Port", "baud rate (9600)"=u32 115200, "stop bits (10: 1 bit)"=w102) -> ("VISA resource name out"=w99:refnum<visa-resource-name>, "error out"=w100:errorcluster)  [unwired: 4 in, 7 out]
  n182 = call "IMAQ Create"("Image Name"="APD 1 Image", "Image Type"=w12) -> ("New Image"=w108:T2)  [unwired: 3 in, 1 out]
  n183 = call "IMAQ Create"("Image Name"="APD 2 Image", "Image Type"=w12) -> ("New Image"=w107:T2)  [unwired: 3 in, 1 out]
  n184 = call "IMAQ Create"("Image Name"="APD 3 Image", "Image Type"=w12) -> ("New Image"=w11:T2)  [unwired: 3 in, 1 out]
  n185 = call "IMAQ Create"("Image Name"="Det. X Image", "Image Type"=w12) -> ("New Image"=w106:T2)  [unwired: 3 in, 1 out]
  n186 = call "IMAQ Create"("Image Name"="Det. Y Image", "Image Type"=w12) -> ("New Image"=w105:T2)  [unwired: 3 in, 1 out]
  n187 = Bundle("New Image"=w108, "New Image"=w107, "New Image"=w11, "New Image"=w106, "New Image"=w105) -> (w104:T22)  [unwired: 1 in]
  n188 = node-c288() -> (w113:T23)  [unwired: 4 in]
  n189 = node-c288(3 ("Processor")) -> (w124:T23)  [unwired: 3 out]
  n190 = node-c288(2 ("Processor")) -> (w126:T23)  [unwired: 3 out]
  n191 = node-c288() -> (w128:T23)  [unwired: 4 out]
  n192 = node-c288(i64 1 ("Period"), 1 ("Processor")) -> (w199:T23)  [unwired: 2 out]
  n193 = timed-loop "Run Scripts, including: stage motion" {
    tunnel: w118 -> [w374]
    tunnel: w117 -> [w375]
    tunnel: [w375] -> w116
    tunnel: [w374] -> w115
    timing: w113 -> [_]
    timing-out: [_] -> w112
    tunnel: w99 -> [w373]
    tunnel: w100 -> [w372]
    tunnel: w71 -> [w369]
    tunnel: w70 -> [w368]
    tunnel: w69 -> [w370]
    tunnel: w68 -> [w371]
    tunnel: w5 -> [w367]
    stop <- w376 stop-if-true
    n194 = node-c288() -> ()  [unwired: 1 in, 1 out]
    n195 = event shown="[5] \"Blue Laser Modluation Mode\": Value Change" {
      selector: _ -> [_ _ _ _ _ _ _ _ _ _ _ _ _ _ _ _ _ _ _ _ _ _ _]
      dyn-events: _ -> [_ _ _ _ _ _ _ _ _ _ _ _ _ _ _ _ _ _ _ _ _ _ _]
      timeout: _ -> [_ _ _ _ _ _ _ _ _ _ _ _ _ _ _ _ _ _ _ _ _ _ _]
      tunnel: ["Set Position" "Move to Position" _ _ _ _ _ _ "Read Harvard" _ _ _ _ _ _ "Got ADig bead" "Force FB Data\nScript" _ "Got DNA bead" "Take Stepping Data" _ "Take Detection Laser\nImage" _] -> _
      tunnel: [_ _ _ _ _ _ _ _ _ _ _ _ _ _ _ _ _ _ _ _ _ _ w1070] -> w376
      tunnel: w374 -> [w394 w402 w415 w445 _ _ _ _ _ w561 w601 w682 w711 w843 w869 _ w905 _ _ _ _ _ _]
      tunnel: w375 -> [w395 w403 w416 w446 _ _ _ _ _ w562 w602 w683 w712 w844 w870 _ w906 _ _ _ _ _ _]
      tunnel: w373 -> [_ _ _ _ _ _ _ _ w546 _ _ _ _ _ _ _ _ _ _ _ _ _ _]
      tunnel: w372 -> [_ _ _ _ _ _ _ _ w545 _ _ _ _ _ _ _ _ _ _ _ _ _ _]
      tunnel: w371 -> [_ _ _ _ _ _ _ _ _ _ _ _ _ _ _ _ _ _ _ _ _ _ _]
      tunnel: w370 -> [_ _ _ _ _ _ _ _ _ _ _ _ _ _ _ _ _ _ _ _ _ _ _]
      tunnel: w369 -> [_ _ _ _ _ _ _ _ _ _ _ _ _ _ _ _ _ _ _ _ _ _ _]
      tunnel: w368 -> [_ _ _ _ _ _ _ _ _ _ _ _ _ _ _ _ _ _ _ _ _ _ _]
      tunnel: w367 -> [_ _ _ _ w473 w501 w525 w536 _ _ _ _ _ _ _ _ _ _ _ _ _ _ w1069]
      event "Set Position", "Set Position 2", "Set Position 3", "Set Position 4", "Set Position 5", "Set Position 1": Value Change {
        n196 = event-data() -> ()  [unwired: 1 in, 5 out]
        n197 = Build Array("Set Position 1", "Set Position 2", "Set Position 3", "Set Position 4", "Set Position 5") -> (w393:bool[])
        n198 = Boolean Array To Number(Boolean array=w393) -> (number=w392:u32)
        n199 = Logarithm Base 2(1:w392) -> (0:w384:dbl)
        n200 = call "Read Stage Position.vi"("error in"=w394, "VISA resource name in"=w395) -> ("Current Position"=w399:cluster{dbl, dbl, dbl}, "error out"=w398:errorcluster)  [unwired: 2 out]
        n201 = Decrement(x="Position") -> (x-1=w382:dbl)
        n202 = Greater Or Equal?(x=w384, y=0.0) -> (x >= y?=w385:bool)
        n203 = Cluster To Array(cluster=w399) -> (array=w396:dbl[])
        n204 = local write "Stage Control Serial Error"(w398) -> ()
        n205 = Select(t=w384, s=w385, f=w382) -> (s? t:f=w381:dbl)
        n206 = Increment(x=w381) -> (x+1=w380:dbl)
        n207 = Build Array (concatenate)(w380, w396) -> (w379:dbl[])
        n208 = Replace Array Subset(array="Saved Stage Positions", new element=w379, index (row)=w381) -> (w397:dbl[][])  [unwired: 1 in]
        n209 = local write "Saved Stage Positions"(w397) -> ()
      }
      event "Move to Position": Value Change {
        n210 = event-data() -> ()  [unwired: 1 in, 5 out]
        n211 = flat-sequence {
          tunnel: w403 -> [w407]
          tunnel: w402 -> [w406]
          frame #0 {
            n212 = local read "Saved Stage Positions"() -> (w409:dbl[][])
            n213 = local read "Position"() -> (w408:dbl)
            n214 = local write "Stage Moving"(TRUE ("Stage Moving")) -> ()
            n215 = call "move to saved stage position.vi"("error in"=w406, "Stage VISA resource name in"=w407, "Position"=w408, "Saved Stage Positions"=w409) -> ("error out"=w405:errorcluster)  [unwired: 1 out]
            n216 = local write "Stage Control Serial Error"(w405) -> ()
          }
          frame #1 {
            n217 = call <vilib>:"Beep.vi"() -> ()  [unwired: 3 in, 9 out]
            n218 = local write "Stage Moving"(FALSE ("Stage Moving")) -> ()
          }
        }
      }
      event "Move Cap. 1 (DNA Bottom)": Value Change {
        n219 = event-data() -> ()  [unwired: 1 in, 5 out]
        n220 = local write "Move Cap. 1 (DNA Bottom)"(FALSE ("Move Cap. 1 (DNA Right)")) -> ()
        n221 = flat-sequence {
          tunnel: w415 -> [w418]
          tunnel: w416 -> [w419]
          tunnel: [w419] -> w413
          tunnel: [w418] -> w412
          tunnel: w413 -> [w421]
          tunnel: w412 -> [w420]
          frame #0 {
            n222 = property on="Sample Channel\nFlow" class="Bool (strict)"("Val(Sgnl)"="Cap 1 Samp Flow ON") -> ()  [unwired: 2 in, 2 out]
          }
          frame #1 {
            n223 = local read "Saved Stage Positions"() -> (w431:dbl[][])
            n224 = local write "Stage Moving"(TRUE ("Stage Moving")) -> ()
            n225 = Array Subset(array=w431, index (row)=0 ("index"), length (row)=1 ("length"), index (col)=1 ("index"), length (col)=3 ("length")) -> (w428:dbl[][])
            n226 = Reshape Array(w428, 3 ("dimension size")) -> (w426:dbl[])
            n227 = Array To Cluster(array=w426) -> (cluster=w425:cluster{"[0]":dbl, "[1]":dbl, "[2]":dbl})
            n228 = call "Set Stage Position.vi"("Position"=w425, "error in"=w420, "VISA resource name in"=w421) -> ("error out"=w424:errorcluster)  [unwired: 2 out]
            n229 = local write "Stage Control Serial Error"(w424) -> ()
          }
          frame #2 {
            n230 = local write "Stage Moving"(FALSE ("Stage Moving")) -> ()
            n231 = case shown="True" "Cap 1 Flow ON" {
              frame False {
              }
              frame True {
                n232 = property on="Inject Pump 1" class="Bool (strict)"("Val(Sgnl)"=TRUE ("Value (Signaling)")) -> ()  [unwired: 2 in, 2 out]
              }
            }
            n233 = call <vilib>:"Beep.vi"() -> ()  [unwired: 3 in, 9 out]
          }
          frame #3 {
            n234 = property on="Sample Channel\nFlow" class="Bool (strict)"("Val(Sgnl)"=FALSE ("Value (Signaling)")) -> ()  [unwired: 2 in, 2 out]
            n235 = local read "Cap. 2 BD T1?\n(ADig T1, DNA T2)"() -> (w438:bool)
            n236 = case shown="True" w438 {
              tunnel: "Cap 1 T ON" -> [w440 w441]
              frame False {
                n237 = property on="Trap 1 (ON/OFF)" class="Bool (strict)"("Val(Sgnl)"=w440) -> ()  [unwired: 2 in, 2 out]
              }
              frame True {
                n238 = property on="Trap 2 (ON/OFF)" class="Bool (strict)"("Val(Sgnl)"=w441) -> ()  [unwired: 2 in, 2 out]
              }
            }
            n239 = property on="Got DNA bead" class="Bool"("Key Focus"=TRUE) -> ()  [unwired: 2 in, 2 out]
          }
        }
      }
